vi "InterpolatePlayPoints.vi"(9 "Total Playing Time (sec)":dbl step=0.1, 10 "Point List":dbl[][][](array[numeric])=[[[60.0, 60.0], [75.0, 75.0]], [[90.0, 90.0], [90.0, 60.0]]], 11 "Ellapsed Time (ms)":u32) -> (2 "Y":u32[](array[numeric]), 3 "X":u32[](array[numeric]))   [LabVIEW 2017, in "AODControl.lvlib"]
uses:
  AODControl.lvlib
  CodifyFrequency(Array).vi
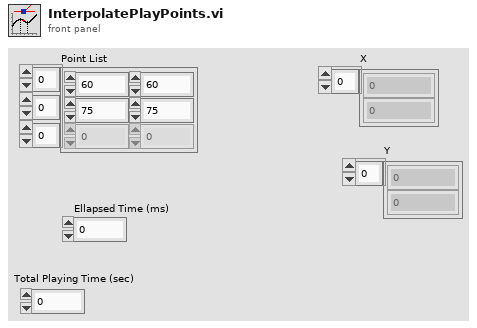
[diagram p1: front panel]
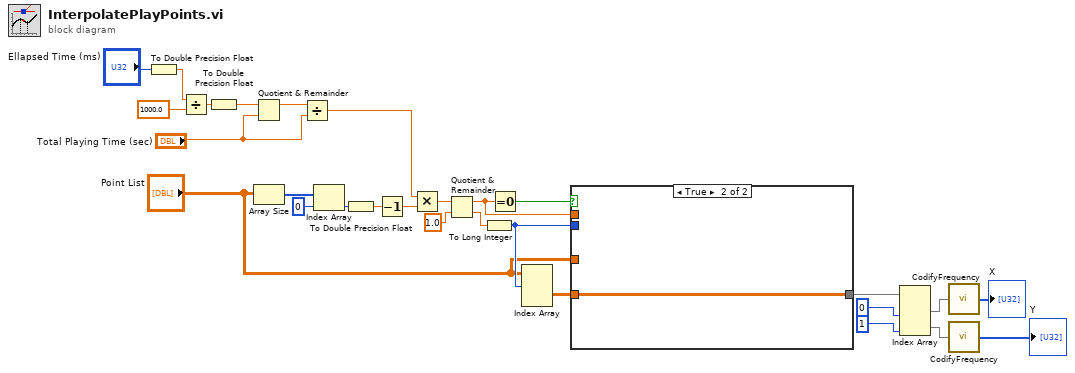
[diagram p0: block diagram]
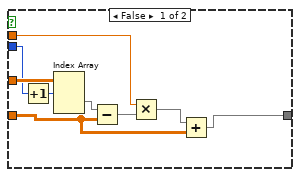
[diagram p2: hidden frame]
diagram:
  n1 = To Double Precision Float(number="Ellapsed Time (ms)") -> (double precision float=w12:dbl)
  n2 = Divide(x=w12, y=1000.0) -> (x/y=w13:dbl)
  n3 = To Double Precision Float(number=w13) -> (double precision float=w3:dbl)
  n4 = Quotient & Remainder(x=w3, y="Total Playing Time (sec)") -> (x-y*floor(x/y)=w1:dbl)  [unwired: 1 out]
  n5 = Array Size(array="Point List") -> (size(s)=w28:i32[])
  n6 = Divide(x=w1, y="Total Playing Time (sec)") -> (x/y=w25:dbl)
  n7 = Index Array(array=w28, index=0) -> (element=w26:i32)
  n8 = To Double Precision Float(number=w26) -> (double precision float=w24:dbl)
  n9 = Decrement(x=w24) -> (x-1=w23:dbl)
  n10 = Multiply(x=w25, y=w23) -> (x*y=w19:dbl)
  n11 = Quotient & Remainder(x=w19, y=1.0) -> (x-y*floor(x/y)=w18:dbl, floor(x/y)=w20:dbl)
  n12 = To Long Integer(number=w20) -> (32bit integer=w17:i32)
  n13 = Equal To 0?(x=w18) -> (x = 0?=w21:bool)
  n14 = Index Array(array="Point List", index (dim 0)=w17) -> (element=w16:dbl[][])  [unwired: 2 in]
  n15 = case shown="True" w21 {
    tunnel: [w29 w38] -> w10
    tunnel: w18 -> [w32 _]
    tunnel: "Point List" -> [w37 _]
    tunnel: w17 -> [w35 _]
    tunnel: w16 -> [w30 w38]
    frame False {
      n16 = Increment(x=w35) -> (x+1=w36:i32)
      n17 = Index Array(array=w37, index (dim 0)=w36) -> (element=w34:dbl[][])  [unwired: 2 in]
      n18 = Subtract(x=w34, y=w30) -> (x-y=w33:dbl[][])
      n19 = Multiply(x=w32, y=w33) -> (x*y=w31:dbl[][])
      n20 = Add(x=w31, y=w30) -> (x+y=w29:dbl[][])
    }
    frame True {
    }
  }
  n21 = Index Array(array=w10, index (col) #1=0 ("index (row)"), index (col) #2=1 ("index (row)")) -> (element #1=w9:dbl[], element #2=w8:dbl[])  [unwired: 2 in]
  n22 = call-poly "CodifyFrequency.vi"("Array"=w9) -> ("Array 2"=→"X":u32[])
  n23 = call-poly "CodifyFrequency.vi"("Array"=w8) -> ("Array 2"=→"Y":u32[])
